vi "svc_Basic Datatype Defaults.vi"() -> (7 "boolean true":bool, 8 "waveform parameters":T1, 9 "boolean false":bool, 10 "empty array of strings":string[](array[string]), 11 "zero I32":i32, 12 "empty string":string, 13 "empty array of DBL":dbl[](array[numeric]), 14 "empty waveform":waveform(dbl), 15 "empty array of waveforms":waveform(dbl)[](array[waveform]), 16 "NaN":dbl=nan, 17 "Inf":dbl=inf, 18 "-Inf":dbl=-inf, 19 "zero DBL":dbl)   [LabVIEW 2017]
uses:
  <vilib>/addons/_NISVFA/_Shared subVIs/Controls/svc_Waveform Parameters.ctl
panel:
  # "do not change default values without\ndue consideration"
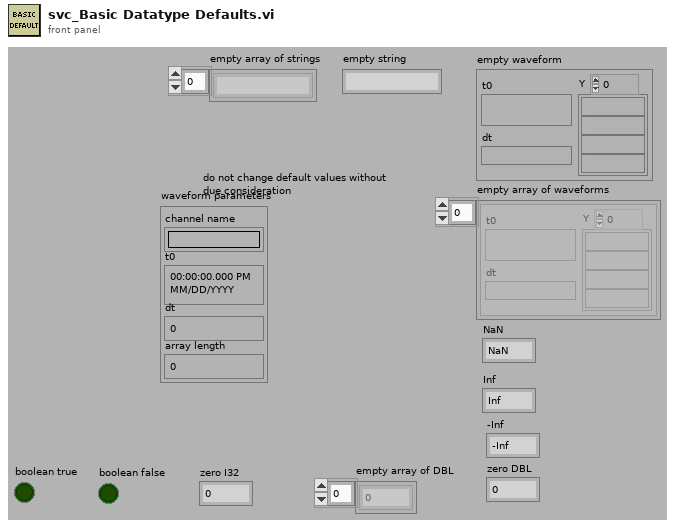
[diagram p1: front panel]
types:
  T1 = typedef "svc_Waveform Parameters.ctl" = cluster{"channel name":string, "t0":timestamp, "dt":dbl, "array length":i32}
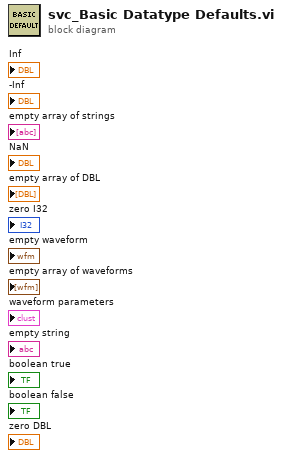
[diagram p0: block diagram]
diagram:
